vi "Reorder DMA values.vi"(6 "Number of signals":u32, 8 "Next Amp array":dbl[](array[numeric]), 9 "Prev Amp array":dbl[](array[numeric]), 10 "Max Amp array":dbl[](array[numeric]), 11 "Max bin array":dbl[](array[numeric])) -> (3 "Ordered array":dbl[](array[numeric]))   [LabVIEW 2014]
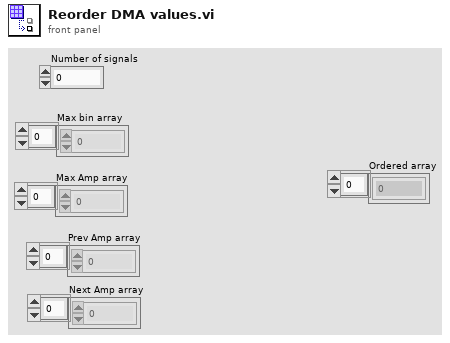
[diagram p1: front panel]
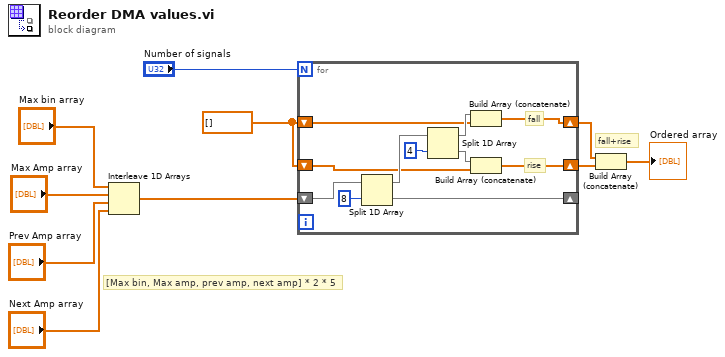
[diagram p0: block diagram]
diagram:
  w10 = dbl[] [] ("first subarray")
  # "fall+rise"
  # "[Max bin, Max amp, prev amp, next amp] * 2 * 5"
  n1 = Interleave 1D Arrays("Max bin array", "Max Amp array", "Prev Amp array", "Next Amp array") -> (w7:dbl[])
  n2 = for {
    N: "Number of signals" -> [_]
    shift-right: [w19] -> _
    shift-left: w7 -> [w21]
    shift-right: [w13] -> w9
    shift-left: w10 -> [w14]
    shift-right: [w11] -> w8
    shift-left: w10 -> [w12]
    # "rise"
    # "fall"
    n3 = Split 1D Array(array=w21, index=8) -> (first subarray=w18:dbl[], second subarray=w19:dbl[])
    n4 = Split 1D Array(array=w18, index=4) -> (first subarray=w15:dbl[], second subarray=w16:dbl[])
    n5 = Build Array (concatenate)(w15, w14) -> (w13:dbl[])
    n6 = Build Array (concatenate)(w16, w12) -> (w11:dbl[])
  }
  n7 = Build Array (concatenate)(w9, w8) -> (→"Ordered array":dbl[])
